vi "WPI_CounterVerifyDigitalSourceOkWithEdgeType.vi"(9 "EdgeType":T5={"Master Mode"=enum."Edge Detection", "UpChannel"=enum."Disabled", "DownChannel"=enum."Disabled", "High/Up"=FALSE}, 10 "Down Source":T1={"DevStatus"={"status"=FALSE, "code"=0, "source"=""}, "AnalogTriggerMode?"=FALSE, "DigitalMode"={"DIO Channel"=enum."Disabled"}, "AnalogTriggerMode"={"AnalogTriggerIndex"=enum."Trig 0", "OutputType"=enum."InWindow"}}, 11 "Up Source":T1={"DevStatus"={"status"=FALSE, "code"=0, "source"=""}, "AnalogTriggerMode?"=FALSE, "DigitalMode"={"DIO Channel"=enum."Disabled"}, "AnalogTriggerMode"={"AnalogTriggerIndex"=enum."Trig 0", "OutputType"=enum."InWindow"}}) -> (0 "error out":errorcluster)   [LabVIEW 2017]
doc: "This software is licensed. Open the labview\\readme\\WPI Robotics Library Open Source License.txt file for more information."
uses:
  <vilib>/Rock Robotics/SystemInterfaces/Counter/FPGA_CounterCtrEdgeDetectionType.ctl
  <vilib>/Rock Robotics/SystemInterfaces/CounterEncoderSourceConvertion/FPGA_CounterEncoderSourceConvertionLVSourceType.ctl
  <vilib>/Rock Robotics/SystemInterfaces/DIO/FPGA_DIODigitalSourceChannel.ctl
  <vilib>/Rock Robotics/SystemInterfaces/AnalogTrigger/FPGA_AnalogTriggerIndex.ctl
  <vilib>/Rock Robotics/SystemInterfaces/AnalogTrigger/FPGA_AnalogTriggerOutType.ctl
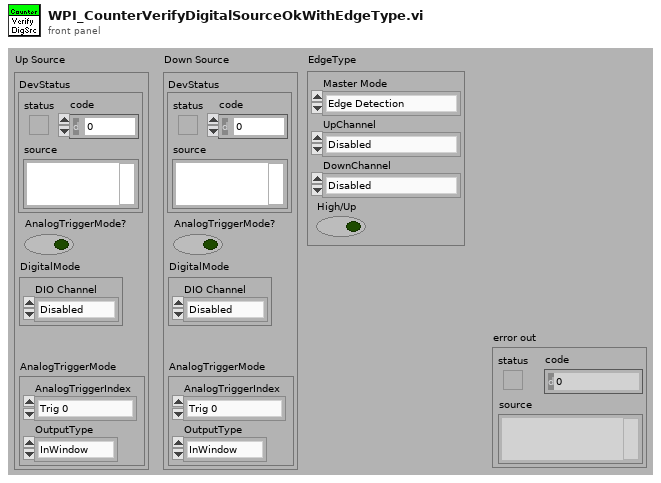
[diagram p1: front panel]
types:
  T1 = typedef "FPGA_CounterEncoderSourceConvertionLVSourceType.ctl" = cluster{"DevStatus":errorcluster, "AnalogTriggerMode?":bool, "DigitalMode":cluster{"DIO Channel":T2}, "AnalogTriggerMode":cluster{"AnalogTriggerIndex":T3, "OutputType":T4}}
  T2 = typedef "FPGA_DIODigitalSourceChannel.ctl" = enum8{"DIO 0", "DIO 1", "DIO 2", "DIO 3", "DIO 4", "DIO 5", "DIO 6", "DIO 7", "DIO 8", "DIO 9", "DIO MXP 0", "DIO MXP 1", "DIO MXP 2", "DIO MXP 3", "DIO MXP 4", "DIO MXP 5", "DIO MXP 6", "DIO MXP 7", "DIO MXP 8", "DIO MXP 9", "DIO MXP 10", "DIO MXP 11", "DIO MXP 12", "DIO MXP 13", "DIO MXP 14", "DIO MXP 15", "Disabled"}
  T3 = typedef "FPGA_AnalogTriggerIndex.ctl" = enum8{"Trig 0", "Trig 1", "Trig 2", "Trig 3", "Trig 4", "Trig 5", "Trig 6", "Trig 7", "Invalid"}
  T4 = typedef "FPGA_AnalogTriggerOutType.ctl" = enum16{"InWindow", "TriggerState", "Rising", "Falling"}
  T5 = typedef "FPGA_CounterCtrEdgeDetectionType.ctl" = cluster{"Master Mode":enum16{"Edge Detection", "Semi Period Mode", "Pulse Length Mode", "External Direction"}, "UpChannel":enum16{"Rising Edge", "Falling Edge", "Raising & Falling Edge", "Disabled"}, "DownChannel":enum16{"Rising Edge", "Falling Edge", "Raising & Falling Edge", "Disabled"}, "High/Up":bool}
  T6 = enum16{"Edge Detection", "Semi Period Mode", "Pulse Length Mode", "External Direction"}
  T7 = enum16{"Rising Edge", "Falling Edge", "Raising & Falling Edge", "Disabled"}
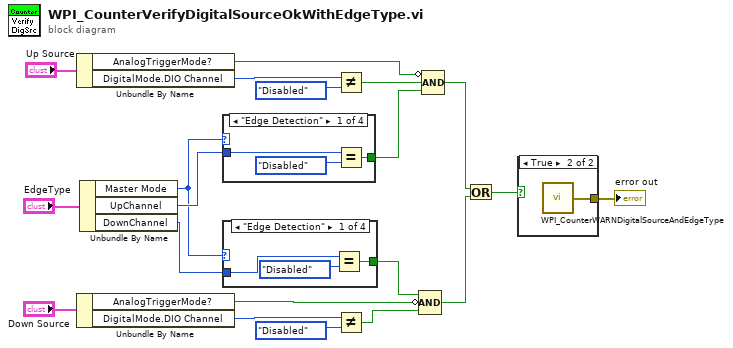
[diagram p0: block diagram]
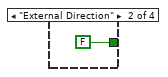
[diagram p3: hidden frame]
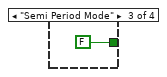
[diagram p4: hidden frame]
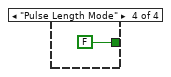
[diagram p5: hidden frame]
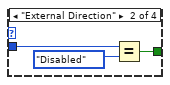
[diagram p6: hidden frame]
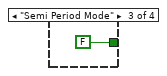
[diagram p7: hidden frame]
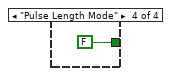
[diagram p8: hidden frame]
diagram:
  n1 = Unbundle By Name("Up Source") -> ("AnalogTriggerMode?"=w17:bool, "DigitalMode.DIO Channel"=w16:T2)
  n2 = Unbundle By Name("Down Source") -> ("AnalogTriggerMode?"=w9:bool, "DigitalMode.DIO Channel"=w8:T2)
  n3 = Unbundle By Name("EdgeType") -> ("Master Mode"=w3:T6, "UpChannel"=w13:T7, "DownChannel"=w7:T7)
  n4 = case shown="\"Edge Detection\"" w3 {
    tunnel: w13 -> [w23 w24 _ _]
    tunnel: [w21 w25 FALSE FALSE] -> w12
    frame "Edge Detection" {
      n5 = Equal?(x=w23, y=T7."Disabled") -> (x = y?=w21:bool)
    }
    frame "External Direction" {
      n6 = Equal?(x=w24, y=T7."Disabled") -> (x = y?=w25:bool)
    }
    frame "Semi Period Mode" {
    }
    frame "Pulse Length Mode" {
    }
  }
  n7 = case shown="\"Edge Detection\"" w3 {
    tunnel: [w31 FALSE FALSE FALSE] -> w4
    tunnel: w7 -> [w29 _ _ _]
    frame "Edge Detection" {
      n8 = Equal?(x=w29, y=T7."Disabled") -> (x = y?=w31:bool)
    }
    frame "External Direction" {
    }
    frame "Semi Period Mode" {
    }
    frame "Pulse Length Mode" {
    }
  }
  n9 = Not Equal?(x=w16, y=FPGA_DIODigitalSourceChannel."Disabled") -> (x != y?=w14:bool)
  n10 = Not Equal?(x=w8, y=FPGA_DIODigitalSourceChannel."Disabled") -> (x != y?=w11:bool)
  n11 = Compound Arithmetic op=AND(w4, invert w9, w11) -> (w5:bool)
  n12 = Compound Arithmetic op=AND(invert w17, w14, w12) -> (w6:bool)
  n13 = Or(x=w6, y=w5) -> (x .or. y?=w1:bool)
  n14 = case shown="True" w1 {
    tunnel: [_ w35] -> w2
    frame False {
    }
    frame True {
      n15 = call <vilib>:"WPI_CounterWARNDigitalSourceAndEdgeType.vi"() -> ("WARNDigitalSourceAndEdgeType"=w35:errorcluster)
    }
  }
  "error out" <- w2
